vi "Post Substeps PWM Generation.vi"(9 "PWM Data in":T1={"Frequency"=1000.0, "Duty Cycle"=0.99, "PWM Action"=enum."PWM Start"}, 10 "Socket No":u16=1, 11 "Sequence Context In":refnum<k7>) -> (0 "error out":errorcluster, 1 "PWM Data out":T1={"Frequency"=1000.0, "Duty Cycle"=0.99, "PWM Action"=enum."PWM Start"}, 3 "Report Text":string)   [LabVIEW 2023, in "LTT_TeststandSteptypes.lvlib"]
doc: "This VI Is Socket Number based AO Data Signal Write Through Q"
uses:
  LTT_TeststandSteptypes.lvlib
  Control/PWM Output Data.ctl
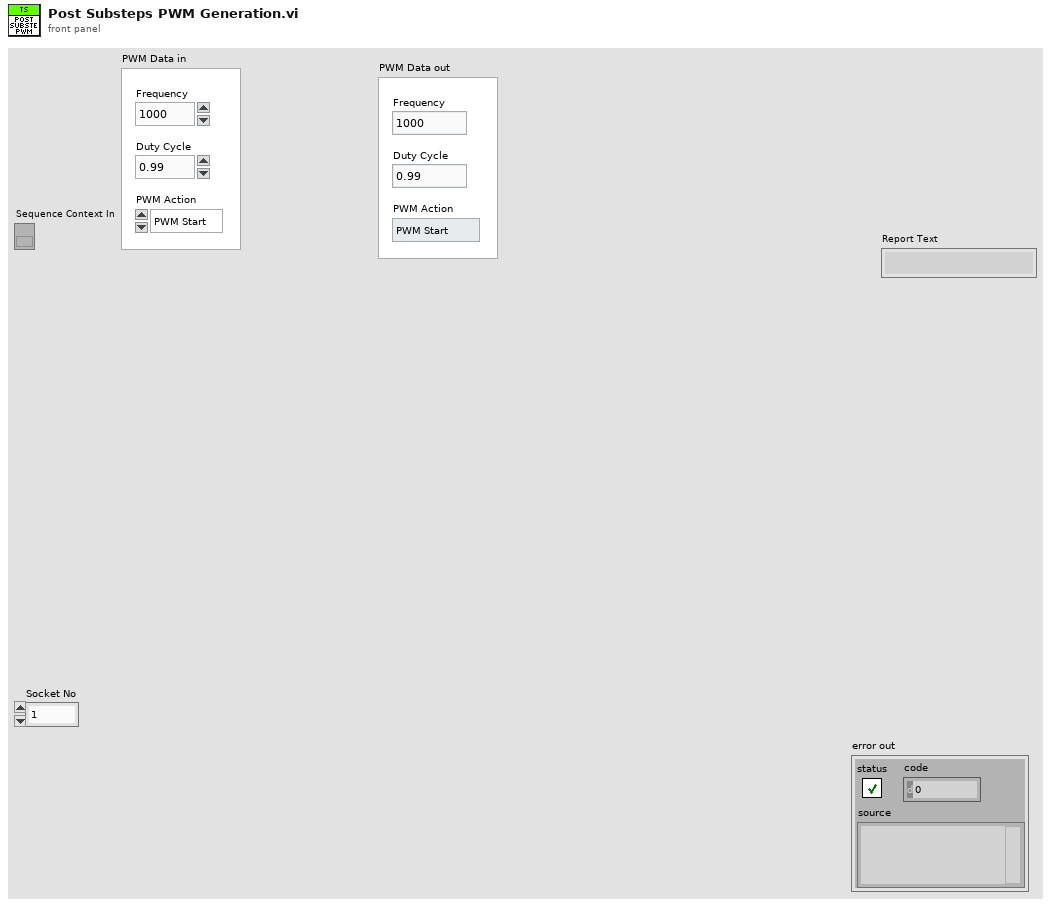
[diagram p1: front panel]
types:
  T1 = typedef "LTT_TeststandSteptypes.lvlib/PWM Output Data.ctl" = cluster{"Frequency":dbl, "Duty Cycle":dbl, "PWM Action":enum16{"PWM Start", "PWM Stop"}}
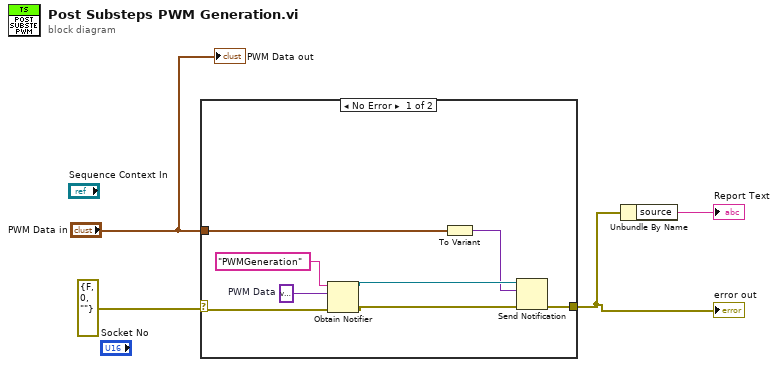
[diagram p0: block diagram]
diagram:
  n1 = case shown="No Error" errorcluster {"status"=FALSE, "code"=0, "source"=""} ("error in") {
    selector: errorcluster {"status"=FALSE, "code"=0, "source"=""} ("error in") -> [w10 w13]
    tunnel: [w12 w13] -> w2
    tunnel: "PWM Data in" -> [w5 _]
    frame No Error {
      w7 = variant  # PWM Data
      n2 = Obtain Notifier(name (unnamed)="PWMGeneration", notification data type=w7, error in (no error)=w10) -> (notifier out=w8:refnum<notifier>, error out=w9:errorcluster)  [unwired: 1 in, 1 out]
      n3 = To Variant(anything=w5) -> (Variant=w6:variant)
      n4 = Send Notification(notification=w6, notifier=w8, error in (no error)=w9) -> (error out=w12:errorcluster)  [unwired: 1 out]
    }
    frame Error {
    }
  }
  "error out" <- w2
  n5 = Unbundle By Name(w2) -> ("source"=→"Report Text":string)
  "PWM Data out" <- "PWM Data in"
